vi "TCP-IP Link.Read Msg with Length Header, 3 digit char.vi"(8 "error in (no error)":errorcluster, 9 "Timeoutms":i32=100, 11 "ConID":refnum<k5>) -> (0 "Error Out":errorcluster, 1 "Timed Out":bool, 2 "data out":string, 3 "ConID Out":refnum<k5>)   [LabVIEW 2024, in "EQMF.lvlib" / "TCP-IP.lvlib"]
uses:
  TCP-IP.lvlib
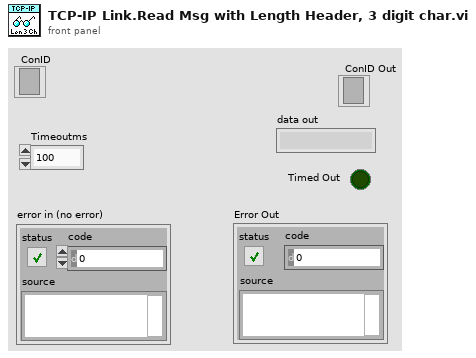
[diagram p1: front panel]
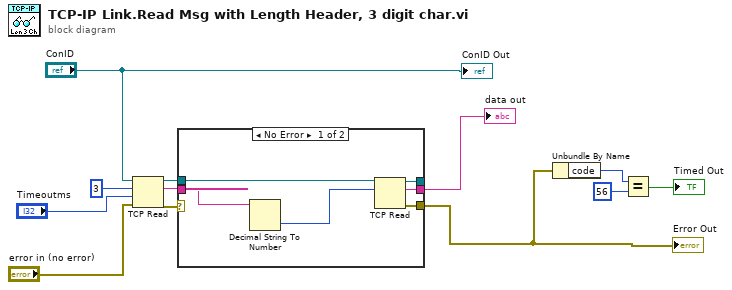
[diagram p0: block diagram]
diagram:
  n1 = TCP Read(connection ID="ConID", bytes to read=3, error in (no error)="error in (no error)", 9:"Timeoutms") -> (connection ID out=w9:refnum<k5>, data out=w11:string, error out=w10:errorcluster)  [unwired: 1 in]
  n2 = case shown="No Error" w10 {
    selector: w10 -> [_ w20]
    tunnel: w11 -> [w14 _]
    tunnel: w9 -> [w18 w19]
    tunnel: [w17 w19] -> _
    tunnel: [w16 _] -> w7
    tunnel: [w15 w20] -> w1
    frame No Error {
      n3 = Decimal String To Number(string=w14) -> (number=w13:i32)  [unwired: 2 in, 1 out]
      n4 = TCP Read(connection ID=w18, bytes to read=w13) -> (connection ID out=w17:refnum<k5>, data out=w16:string, error out=w15:errorcluster)  [unwired: 3 in]
    }
    frame Error {
    }
  }
  "Error Out" <- w1
  "data out" <- w7
  n5 = Unbundle By Name(w1) -> ("code"=w4:i32)
  n6 = Equal?(x=w4, y=56) -> (x = y?=→"Timed Out":bool)
  "ConID Out" <- "ConID"
